vi "TRO.vi"(0 "System no.":i32=1 min=1 max=4 step=1, 2 "TriggerOut to command":string[](array[string]), 3 "Trigger status":bool[](array[boolean]), 5 "error in":errorcluster) -> (19 "error out":errorcluster)   [LabVIEW 2020]
doc: "Enables or disables the trigger output mode which was set with CTO. Do not use DIO on output lines for which the trigger output is activated with TRO.\n\nC-702: TriggerOut to command can be 1 to 8.\n\nC-843: TriggerOut to command can be 1 to 4 (4-axis card) or 2 (2-axis card).\n\nC-866: TriggerOut to command can be 1.\n\nC-867, C-877: Check controller user manual for available output trigger numbers.\n\nC-413, C-884 , E-871, E-873, E-874 : Check controller user manual for available output trigger numbers.\n\nMercury: TriggerOut to command can be 1 to N (N: number of connected axes, if supported by corresponding Mercury firmware).\n\nMercury_GCS: Check Mercury user manual for available output trigger numbers."
panel:
  # "Enables or disables the TRrigger Output mode which was set with CTO."
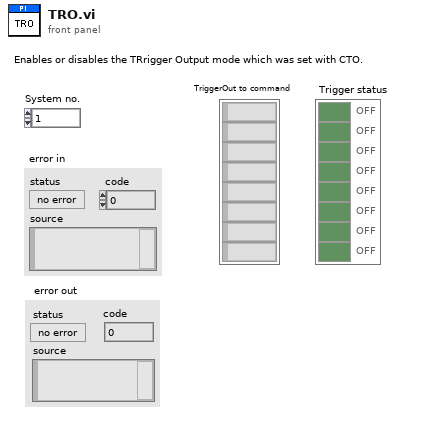
[diagram p1: front panel]
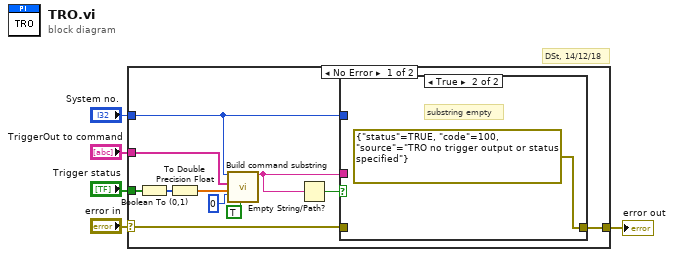
[diagram p0: block diagram]
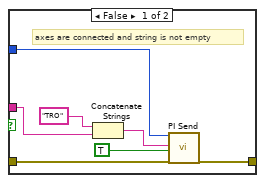
[diagram p2: hidden frame]
diagram:
  # "DSt, 14/12/18"
  n1 = case shown="No Error" "error in" {
    selector: "error in" -> [w6 w25]
    tunnel: [w16 w25] -> w5
    tunnel: "System no." -> [w11 _]
    tunnel: "TriggerOut to command" -> [w15 _]
    tunnel: "Trigger status" -> [w14 _]
    frame No Error {
      n2 = Boolean To (0,1)(Boolean=w14) -> (0, 1=w13:i16[])
      n3 = To Double Precision Float(number=w13) -> (double precision float=w12:dbl[])
      n4 = call "Build command substring.vi"("System no."=w11, "Affected axes"=w15, "Parameters"=w12, "No. of digits"=i16 0 ("No.of digits"), "With space?"=TRUE) -> ("Command substring"=w8:string)  [unwired: 2 in, 12 out]
      n5 = Empty String/Path?(string/path=w8) -> (empty?=w7:bool)
      n6 = case shown="True" w7 {
        tunnel: w8 -> [w22 _]
        tunnel: [w18 errorcluster {"status"=TRUE, "code"=100, "source"="TRO no trigger output or status specified"} ("error out")] -> w16
        tunnel: w6 -> [w19 _]
        tunnel: w11 -> [w17 _]
        frame False {
          # "axes are connected and string is not empty"
          n7 = Concatenate Strings("TRO", w22) -> (w20:string)
          n8 = call "PI Send.vi"("System no."=w17, "String to send"=w20, "Attach termination char.?"=TRUE ("Attach Linefeed?"), "error in"=w19) -> ("error out"=w18:errorcluster)  [unwired: 2 in, 13 out]
        }
        frame True {
          # "substring empty"
        }
      }
    }
    frame Error {
    }
  }
  "error out" <- w5
